vi "Program09.vi"() -> ()   [LabVIEW 2020]
panel:
  out "LED 2":bool
  out "LED1":bool
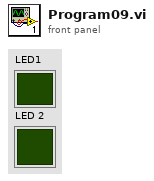
[diagram p1: front panel]
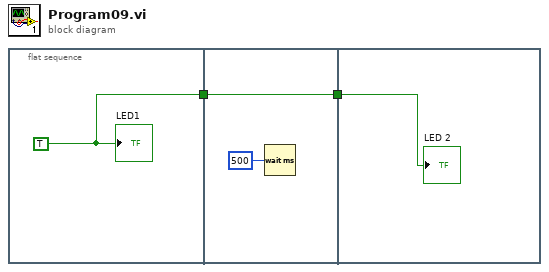
[diagram p0: block diagram]
diagram:
  n1 = flat-sequence {
    tunnel: [w3] -> w1
    tunnel: [w4] -> w2
    tunnel: w1 -> [w4]
    tunnel: w2 -> [w6]
    frame #0 {
      w3 = TRUE
      "LED1" <- w3
    }
    frame #1 {
      n2 = Wait (ms)(milliseconds to wait=u32 500) -> ()  [unwired: 1 out]
    }
    frame #2 {
      "LED 2" <- w6
    }
  }
